vi "CRYAPI FRAME.vi"(4 "tFrame_In":T2, 6 "tSpliter":T3, 8 "tFrame":T2, 9 "sData":string, 10 "nData":i32, 11 "sAction":string) -> (0 "nData_Out":i32, 1 "sData_Out":string, 2 "tSpliter_Out":T3, 3 "tFrame_Out":T2)   [LabVIEW 2013]
uses:
  <vilib>/Utility/miscctls.llb/LVRectTypeDef.ctl
  CRYMain Sub Window Global.vi
  CRYProject/CRYProject Editor Global.vi
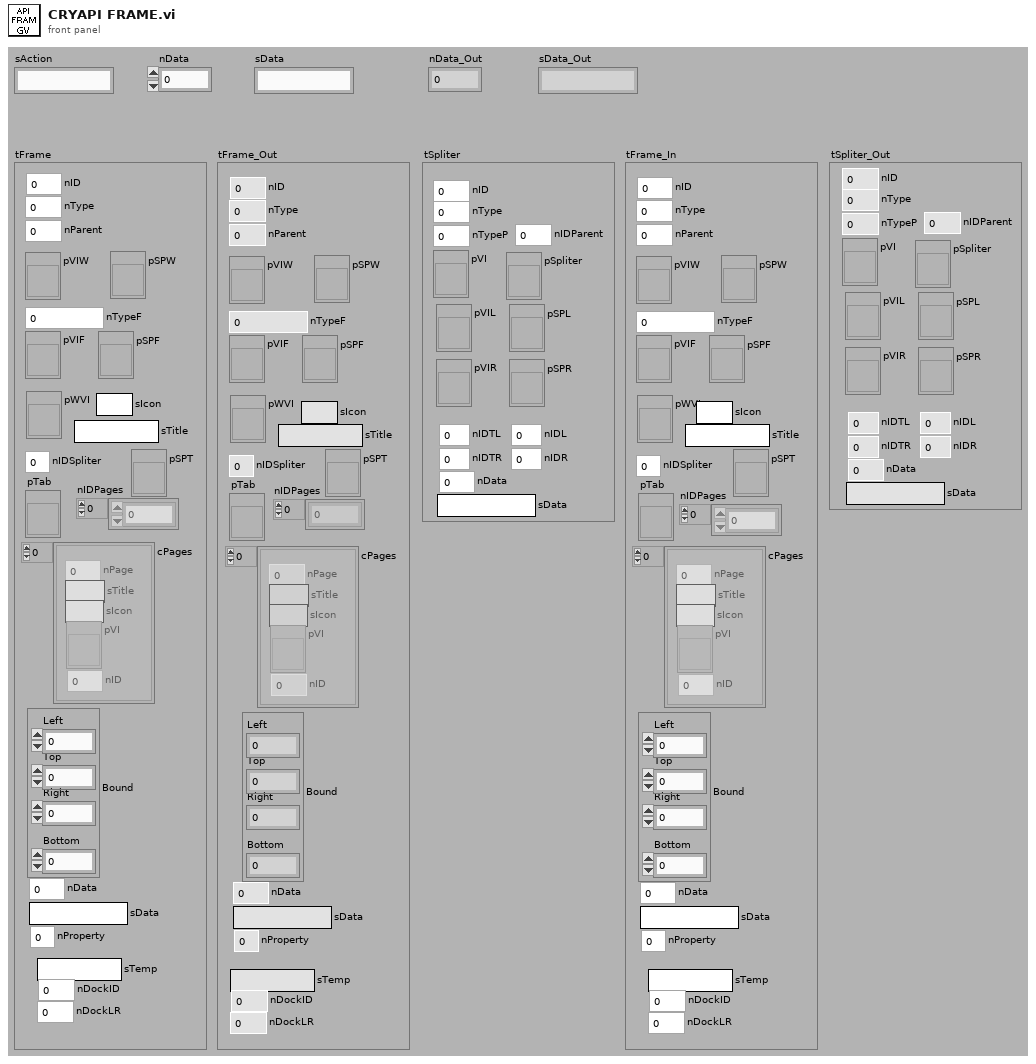
[diagram p1: front panel]
types:
  T1 = typedef "LVRectTypeDef.ctl" = cluster{"Left":i16, "Top":i16, "Right":i16, "Bottom":i16}
  T2 = cluster{"nType":i32, "nParent":i32, "pVIW":refnum<vi>, "pSPW":refnum<vi>, "nTypeF":i32, "pVIF":refnum<vi>, "pSPF":refnum<vi>, "nIDSpliter":i32, "nProperty":i32, "Bound":T1, "nID":i32, "nData":i32, "sData":string, "pWVI":refnum<vi>, "sTitle":string, "cPages":cluster{"nPage":i32, "sTitle":string, "sIcon":string, "pVI":refnum<vi>, "nID":i32}[], "pTab":refnum<vi>, "nIDPages":i32[], "pSPT":refnum<vi>, "sTemp":string, "nDockID":i32, "nDockLR":i32, "sIcon":string}
  T3 = cluster{"nType":i32, "nTypeP":i32, "pVI":refnum<vi>, "pSpliter":refnum<vi>, "pSPL":refnum<vi>, "pVIL":refnum<vi>, "pSPR":refnum<vi>, "pVIR":refnum<vi>, "nIDTL":i32, "nIDL":i32, "nIDTR":i32, "nIDR":i32, "nID":i32, "nIDParent":i32, "nData":i32, "sData":string}
  T4 = cluster{"nPage":i32, "sTitle":string, "sIcon":string, "pVI":refnum<vi>, "nID":i32}[]
  T5 = cluster{"nID":i32, "sTiltle":string, "pVI":refnum<vi>, "pSP":refnum<vi>, "pTab":refnum<vi>, "pSPT":refnum<vi>, "nWinType":i32, "sIcon":string}
  T6 = cluster{"nID":i32[], "Frame":cluster{"nType":i32, "nParent":i32, "pVIW":refnum<vi>, "pSPW":refnum<vi>, "nTypeF":i32, "pVIF":refnum<vi>, "pSPF":refnum<vi>, "nIDSpliter":i32, "nProperty":i32, "Bound":T1, "nID":i32, "nData":i32, "sData":string, "pWVI":refnum<vi>, "sTitle":string, "cPages":cluster{"nPage":i32, "sTitle":string, "sIcon":string, "pVI":refnum<vi>, "nID":i32}[], "pTab":refnum<vi>, "nIDPages":i32[], "pSPT":refnum<vi>, "sTemp":string, "nDockID":i32, "nDockLR":i32, "sIcon":string}[]}
  T7 = cluster{"nType":i32, "nParent":i32, "pVIW":refnum<vi>, "pSPW":refnum<vi>, "nTypeF":i32, "pVIF":refnum<vi>, "pSPF":refnum<vi>, "nIDSpliter":i32, "nProperty":i32, "Bound":T1, "nID":i32, "nData":i32, "sData":string, "pWVI":refnum<vi>, "sTitle":string, "cPages":cluster{"nPage":i32, "sTitle":string, "sIcon":string, "pVI":refnum<vi>, "nID":i32}[], "pTab":refnum<vi>, "nIDPages":i32[], "pSPT":refnum<vi>, "sTemp":string, "nDockID":i32, "nDockLR":i32, "sIcon":string}[]
  T8 = typedef "CRYTS.ctl" = cluster{"No.TS":u16, "TS File Path":path, "TS Name":string, "EditStepName":string, "Steps":T9[], "New State":bool, "Change State":bool, "Flattened CurveLib Data":string, "Document Data":string, "EditStepNo":u16, "Operator Start File":string, "Sequence Type":string, "Sequence Language":string}
  T9 = typedef "CRYStep.ctl" = cluster{"No.VI":i32, "Category":string, "StepName":string, "Seq setup flattened":string, "Comment":string, "Steps config.":bool[], "Jump config":i32[], "Start":dbl, "Increment":dbl, "Name":string, "Unit":string, "Y data":u16, "Y prefix":string, "Y dB ref":dbl, "Y unit":string, "Repeat State Array":cluster{"Start":dbl, "Increment":dbl, "Count":i32, "Num":i32}[]}
  T10 = typedef "LVPointTypeDef.ctl" = cluster{"Horizontal":i16, "Vertical":i16}
  T11 = typedef "LVBoundsTypeDef.ctl" = cluster{"Width":u32, "Height":u32}
  T12 = cluster{"nPage":i32, "sTitle":string, "sIcon":string, "pVI":refnum<vi>, "nID":i32}
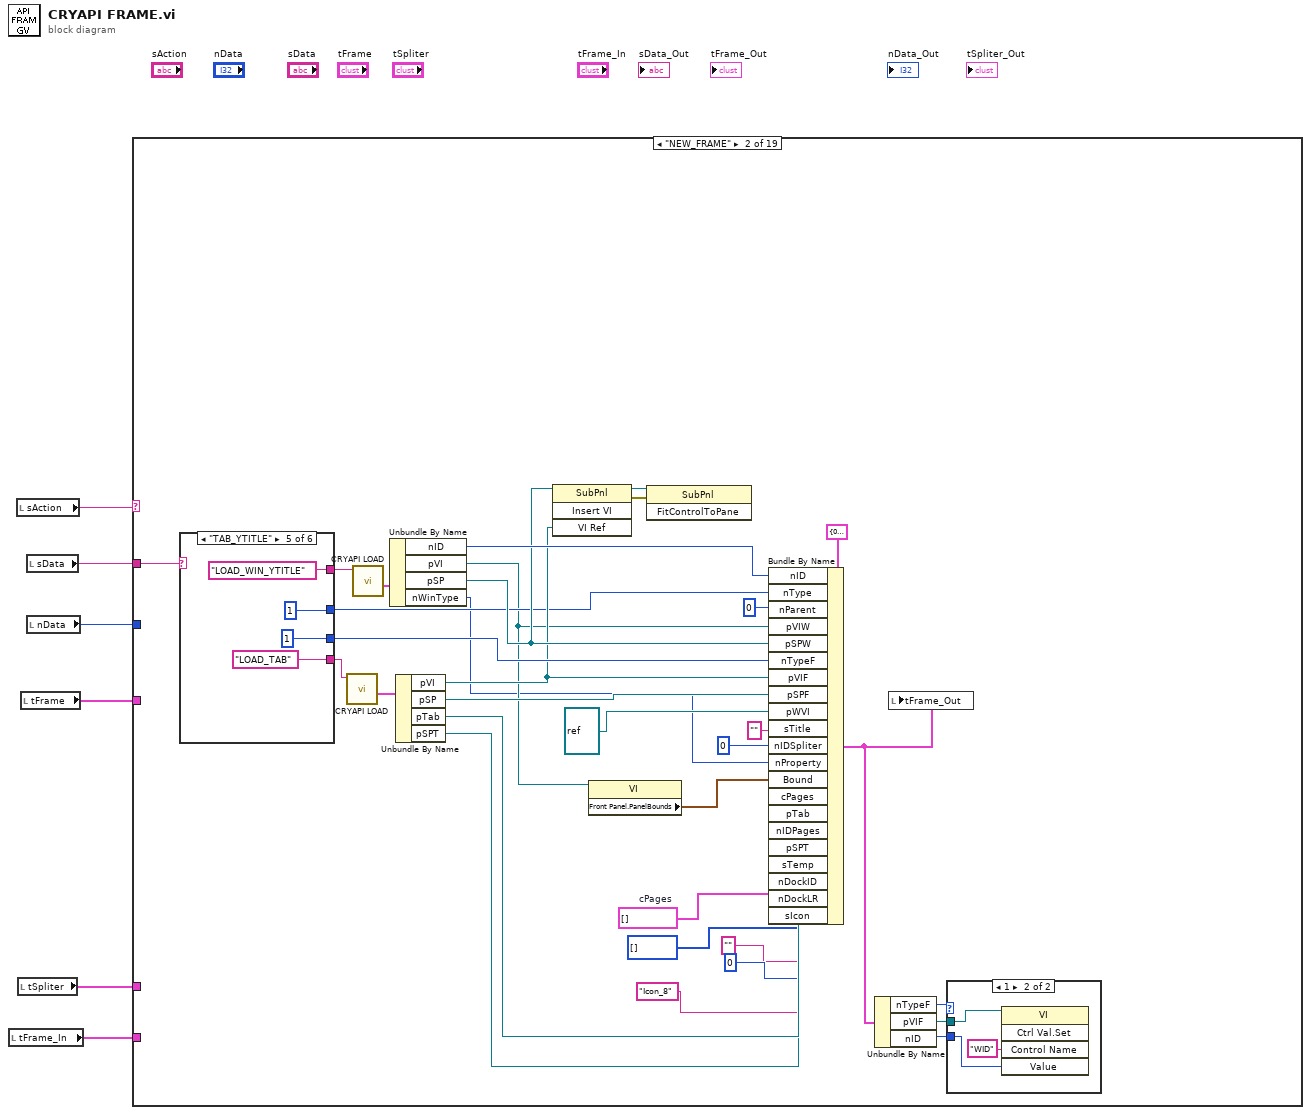
[diagram p0: block diagram]
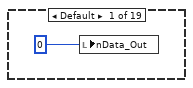
[diagram p2: hidden frame]
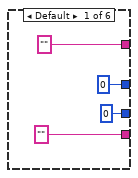
[diagram p4: hidden frame]
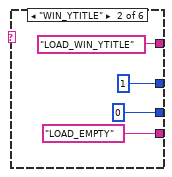
[diagram p5: hidden frame]
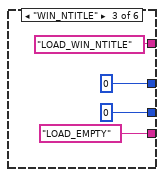
[diagram p6: hidden frame]
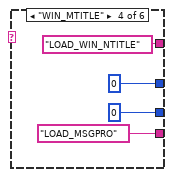
[diagram p7: hidden frame]
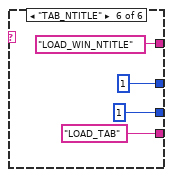
[diagram p8: hidden frame]
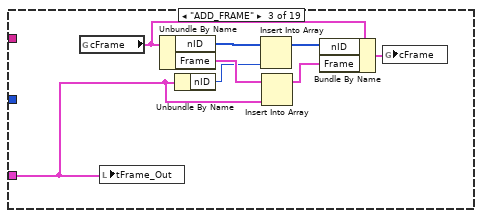
[diagram p9: hidden frame]
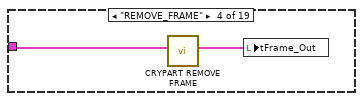
[diagram p10: hidden frame]
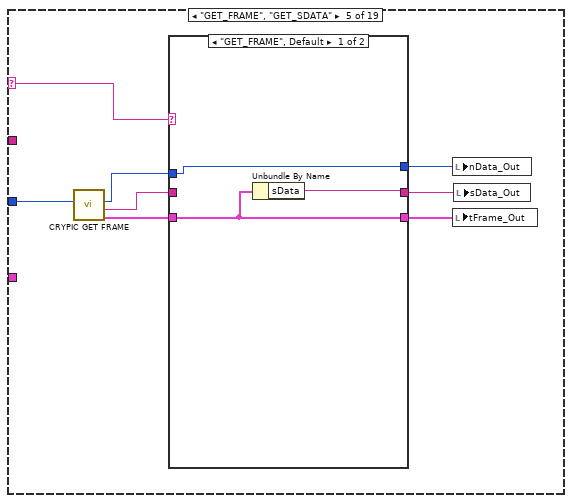
[diagram p11: hidden frame]
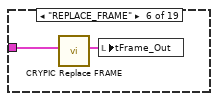
[diagram p13: hidden frame]
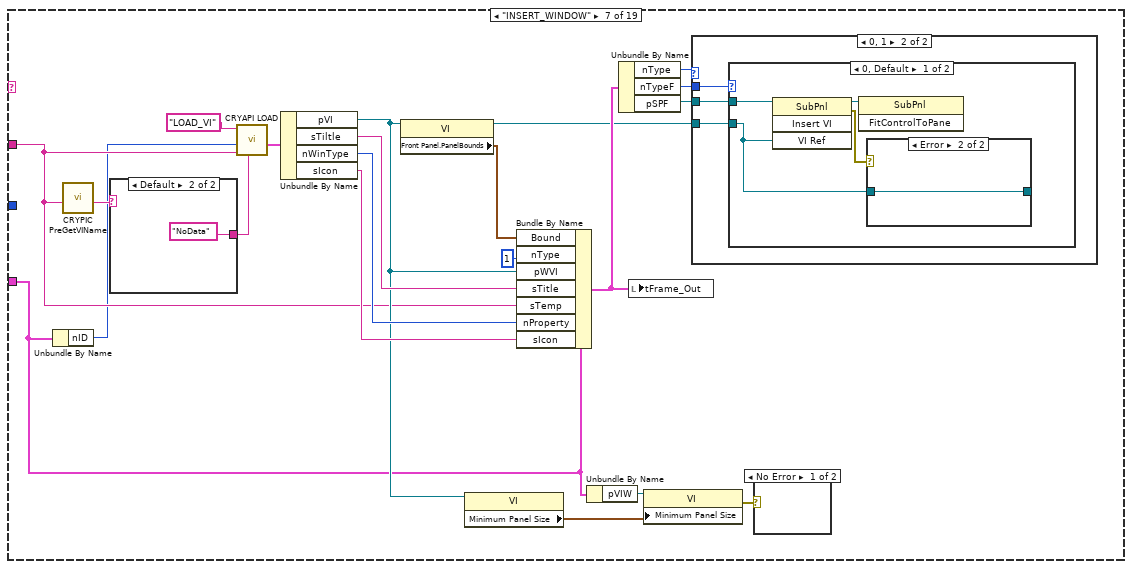
[diagram p14: hidden frame]
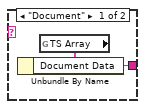
[diagram p16: hidden frame]
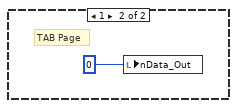
[diagram p19: hidden frame]
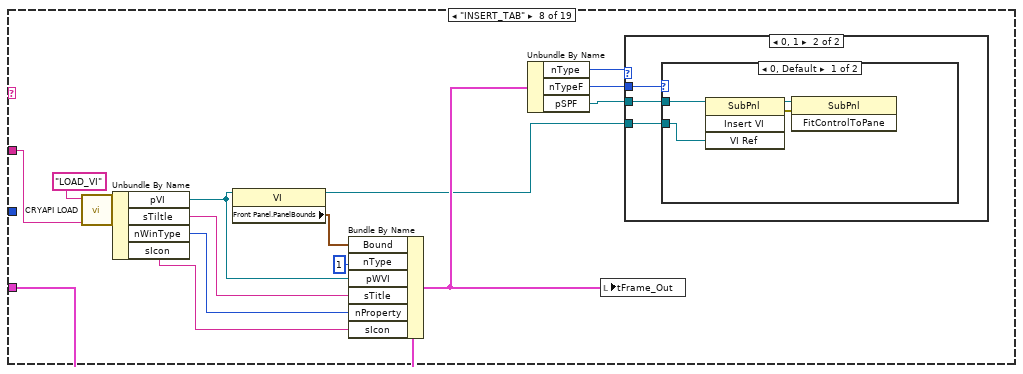
[diagram p20: hidden frame]
diagram:
  n1 = local read "tFrame_In"() -> (w1:T2)
  n2 = local read "sAction"() -> (w6:string)
  n3 = local read "tSpliter"() -> (w2:T3)
  n4 = local read "tFrame"() -> (w3:T2)
  n5 = local read "sData"() -> (w4:string)
  n6 = local read "nData"() -> (w5:i32)
  n7 = case shown="\"NEW_FRAME\"" w6 {
    selector: w6 -> [_ _ _ _ w80 _ _ _ _ w174 _ _ _ w378 w451 _ w569 _ _]
    tunnel: w5 -> [_ _ _ _ w84 _ _ _ _ _ _ _ _ _ _ w534 w568 _ _]
    tunnel: w4 -> [_ w19 _ _ _ _ w95 w139 _ _ _ _ _ _ _ _ w574 _ _]
    tunnel: w3 -> [_ _ w67 w76 _ w91 w94 w127 w163 w175 w300 w320 w348 w377 w452 w526 _ w628 w641]
    tunnel: w2 -> [_ _ _ _ _ _ _ _ w157 _ _ w319 w344 _ _ _ _ _ _]
    tunnel: w1 -> [_ _ _ _ _ _ _ _ _ w168 w302 _ _ _ _ _ _ _ _]
    frame Default {
      n8 = local write "nData_Out"(0 ("nData_Out")) -> ()
    }
    frame "NEW_FRAME" {
      w13 = 0 ("nIDChain")
      w26 = T4 []  # cPages
      n9 = case shown="\"TAB_YTITLE\"" w19 {
        tunnel: ["" ("sAction") "LOAD_WIN_YTITLE" ("sAction") "LOAD_WIN_NTITLE" ("sAction") "LOAD_WIN_NTITLE" ("sAction") "LOAD_WIN_YTITLE" ("sAction") "LOAD_WIN_NTITLE" ("sAction")] -> w12
        tunnel: ["" ("sAction") "LOAD_EMPTY" ("sAction") "LOAD_EMPTY" ("sAction") "LOAD_MSGPRO" ("sAction") "LOAD_TAB" ("sAction") "LOAD_TAB" ("sAction")] -> w18
        tunnel: [0 ("nTypeF") 0 ("nTypeF") 0 ("nTypeF") 0 ("nTypeF") 1 ("nTypeF") 1 ("nTypeF")] -> w34
        tunnel: [0 ("nTypeF") 1 ("nTypeF") 0 ("nTypeF") 0 ("nTypeF") 1 ("nTypeF") 1 ("nTypeF")] -> w29
        frame Default {
        }
        frame "WIN_YTITLE" {
        }
        frame "WIN_NTITLE" {
        }
        frame "WIN_MTITLE" {
        }
        frame "TAB_YTITLE" {
        }
        frame "TAB_NTITLE" {
        }
      }
      n10 = call "CRYAPI LOAD.vi"("sAction"=w18) -> ("tWindow_Out"=w17:T5)  [unwired: 5 in, 5 out]
      n11 = call "CRYAPI LOAD.vi"("sAction"=w12) -> ("tWindow_Out"=w37:T5)  [unwired: 5 in, 5 out]
      n12 = Unbundle By Name(w37) -> ("nID"=w36:i32, "pVI"=w15:refnum<vi>, "pSP"=w33:refnum<vi>, "nWinType"=w11:i32)
      n13 = Unbundle By Name(w17) -> ("pVI"=w32:refnum<vi>, "pSP"=w35:refnum<vi>, "pTab"=w25:refnum<vi>, "pSPT"=w16:refnum<vi>)
      n14 = invoke class="SubPnl" method="Insert VI"(reference=w33, "VI Ref"=w32) -> (reference out=w31:refnum<vi>, error out=w30:errorcluster)  [unwired: 2 in, 2 out]
      n15 = property class="VI"(reference=w15) -> ("Front Panel.PanelBounds"=w14:T1)  [unwired: 1 in, 2 out]
      n16 = invoke class="SubPnl" method="FitControlToPane"(reference=w31, error in=w30) -> ()  [unwired: 1 in, 3 out]
      n17 = Bundle By Name(cluster=T2 {"nType"=0, "nParent"=0, "pVIW"=refnum, "pSPW"=refnum, "nTypeF"=0, "pVIF"=refnum, "pSPF"=refnum, "nIDSpliter"=0, "nProperty"=0, "Bound"={"Left"=100, "Top"=100, "Right"=200, "Bottom"=200}, "nID"=0, "nData"=0, "sData"="", "pWVI"=refnum, "sTitle"="", "cPages"=[], "pTab"=refnum, "nIDPages"=[], "pSPT"=refnum, "sTemp"="", "nDockID"=0, "nDockLR"=0, "sIcon"=""} ("tFrame_Out"), "nID"=w36, "nType"=w29, "nParent"=0, "pVIW"=w15, "pSPW"=w33, "nTypeF"=w34, "pVIF"=w32, "pSPF"=w35, "pWVI"=refnum<vi> refnum, "sTitle"="", "nIDSpliter"=0 ("nIDChain"), "nProperty"=w11, "Bound"=w14, "cPages"=w26, "pTab"=w25, "nIDPages"=i32[] [], "pSPT"=w16, "sTemp"="", "nDockID"=w13, "nDockLR"=w13, "sIcon"="Icon_8") -> (w24:T2)
      n18 = Unbundle By Name(w24) -> ("nTypeF"=w23:i32, "pVIF"=w22:refnum<vi>, "nID"=w21:i32)
      n19 = local write "tFrame_Out"(w24) -> ()
      n20 = case shown="1" w23 {
        tunnel: w22 -> [_ w42]
        tunnel: w21 -> [_ w40]
        frame Default {
        }
        frame 1 {
          n21 = invoke class="VI" method="Ctrl Val.Set"(reference=w42, "Control Name"="WID", "Value"=w40) -> ()  [unwired: 2 in, 5 out]
        }
      }
    }
    frame "ADD_FRAME" {
      n22 = global read "CRYMain Sub Window Global.vi" "cFrame"() -> (w71:T6)
      n23 = local write "tFrame_Out"(w67) -> ()
      n24 = Unbundle By Name(w71) -> ("nID"=w74:i32[], "Frame"=w73:T7)
      n25 = Unbundle By Name(w67) -> ("nID"=w72:i32)
      n26 = Insert Into Array(array=w74, new element=w72) -> (w70:i32[])  [unwired: 1 in]
      n27 = Insert Into Array(array=w73, new element=w67) -> (w69:T7)  [unwired: 1 in]
      n28 = Bundle By Name(cluster=w71, "nID"=w70, "Frame"=w69) -> (w68:T6)
      n29 = global write "CRYMain Sub Window Global.vi" "cFrame"(w68) -> ()
    }
    frame "REMOVE_FRAME" {
      n30 = call "CRYPART REMOVE FRAME.vi"("tFrame"=w76) -> ("tFrame_Out"=w75:T2)  [unwired: 10 in]
      n31 = local write "tFrame_Out"(w75) -> ()
    }
    frame "GET_FRAME", "GET_SDATA" {
      n32 = call "CRYPIC GET FRAME.vi"("nID"=w84) -> ("tFrame_Out"=w81:T2, "sData_Out"=w82:string, "nID_Out"=w83:i32)  [unwired: 8 in]
      n33 = case shown="\"GET_FRAME\", Default" w80 {
        tunnel: w83 -> [w87 w90]
        tunnel: w82 -> [_ w88]
        tunnel: w81 -> [w86 w89]
        tunnel: [w87 w90] -> w79
        tunnel: [w85 w88] -> w78
        tunnel: [w86 w89] -> w77
        frame "GET_FRAME", Default {
          n34 = Unbundle By Name(w86) -> ("sData"=w85:string)
        }
        frame "GET_SDATA" {
        }
      }
      n35 = local write "nData_Out"(w79) -> ()
      n36 = local write "tFrame_Out"(w77) -> ()
      n37 = local write "sData_Out"(w78) -> ()
    }
    frame "REPLACE_FRAME" {
      n38 = call "CRYPIC Replace FRAME.vi"("tFrame"=w91) -> ("tFrame_Out"=w92:T2)  [unwired: 10 in]
      n39 = local write "tFrame_Out"(w92) -> ()
    }
    frame "INSERT_WINDOW" {
      n40 = Unbundle By Name(w94) -> ("nID"=w93:i32)
      n41 = call "CRYPIC PreGetVIName.vi"("sVIName"=w95) -> ("sVIName_Out"=w96:string)  [unwired: 9 in, 1 out]
      n42 = case shown="Default" w96 {
        tunnel: [w114 "NoData" ("sOption")] -> w101
        frame "Document" {
          n43 = global read "CRYProject Editor Global.vi" "TS Array"() -> (w115:T8)
          n44 = Unbundle By Name(w115) -> ("Document Data"=w114:string)
        }
        frame Default {
        }
      }
      n45 = call "CRYAPI LOAD.vi"("sOption"=w101, "sData"=w95, "nData"=w93, "sAction"="LOAD_VI") -> ("tWindow_Out"=w103:T5)  [unwired: 2 in, 5 out]
      n46 = Unbundle By Name(w103) -> ("pVI"=w98:refnum<vi>, "sTiltle"=w106:string, "nWinType"=w105:i32, "sIcon"=w104:string)
      n47 = property class="VI"(reference=w98) -> (reference out=w109:refnum<vi>, "Front Panel.PanelBounds"=w112:T1)  [unwired: 1 in, 1 out]
      n48 = property class="VI"(reference=w98) -> ("Minimum Panel Size"=w99:T10)  [unwired: 1 in, 2 out]
      n49 = Bundle By Name(cluster=w94, "Bound"=w112, "nType"=1, "pWVI"=w98, "sTitle"=w106, "sTemp"=w95, "nProperty"=w105, "sIcon"=w104) -> (w111:T2)
      n50 = Unbundle By Name(w94) -> ("pVIW"=w100:refnum<vi>)
      n51 = Unbundle By Name(w111) -> ("nType"=w110:i32, "nTypeF"=w108:i32, "pSPF"=w107:refnum<vi>)
      n52 = local write "tFrame_Out"(w111) -> ()
      n53 = property class="VI"(reference=w100, "Minimum Panel Size"=w99) -> (error out=w97:errorcluster)  [unwired: 1 in, 1 out]
      n54 = case shown="0, 1" w110 {
        tunnel: w109 -> [_ w117]
        tunnel: w108 -> [_ w119]
        tunnel: w107 -> [_ w118]
        frame Default {
        }
        frame 0, 1 {
          n55 = case shown="0, Default" w119 {
            tunnel: w118 -> [w122 _]
            tunnel: w117 -> [w120 _]
            frame 0, Default {
              n56 = invoke class="SubPnl" method="Insert VI"(reference=w122, "VI Ref"=w120) -> (reference out=w123:refnum<vi>, error out=w121:errorcluster)  [unwired: 2 in, 2 out]
              n57 = invoke class="SubPnl" method="FitControlToPane"(reference=w123) -> ()  [unwired: 2 in, 3 out]
              n58 = case shown="Error" w121 {
                tunnel: [w124 w125] -> _
                tunnel: w120 -> [w124 w125]
                frame No Error {
                }
                frame Error {
                }
              }
            }
            frame 1 {
              # "TAB Page"
              n59 = local write "nData_Out"(0 ("nData_Out")) -> ()
            }
          }
        }
      }
      n60 = case shown="No Error" w97 {
        frame No Error {
        }
        frame Error {
        }
      }
    }
    frame "INSERT_TAB" {
      n61 = call "CRYAPI LOAD.vi"("sData"=w139, "sAction"="LOAD_VI") -> ("tWindow_Out"=w140:T5)  [unwired: 4 in, 5 out]
      n62 = Unbundle By Name(w140) -> ("pVI"=w132:refnum<vi>, "sTiltle"=w131:string, "nWinType"=w130:i32, "sIcon"=w129:string)
      n63 = property class="VI"(reference=w132) -> (reference out=w128:refnum<vi>, "Front Panel.PanelBounds"=w137:T1)  [unwired: 1 in, 1 out]
      n64 = Bundle By Name(cluster=w127, "Bound"=w137, "nType"=1, "pWVI"=w132, "sTitle"=w131, "nProperty"=w130, "sIcon"=w129) -> (w136:T2)
      n65 = Unbundle By Name(w136) -> ("nType"=w135:i32, "nTypeF"=w134:i32, "pSPF"=w133:refnum<vi>)
      n66 = local write "tFrame_Out"(w136) -> ()
      n67 = case shown="0, 1" w135 {
        tunnel: w128 -> [_ w142]
        tunnel: w134 -> [_ w144]
        tunnel: w133 -> [_ w143]
        frame Default {
        }
        frame 0, 1 {
          n68 = case shown="0, Default" w144 {
            tunnel: w143 -> [w146 _]
            tunnel: w142 -> [w145 _]
            frame 0, Default {
              n69 = invoke class="SubPnl" method="Insert VI"(reference=w146, "VI Ref"=w145) -> (reference out=w148:refnum<vi>, error out=w147:errorcluster)  [unwired: 2 in, 2 out]
              n70 = invoke class="SubPnl" method="FitControlToPane"(reference=w148, error in=w147) -> ()  [unwired: 1 in, 3 out]
            }
            frame 1 {
              # "TAB Page"
              n71 = local write "nData_Out"(0 ("nData_Out")) -> ()
            }
          }
        }
      }
    }
    frame "INSERT_SPLITER" {
      n72 = Unbundle By Name(w163) -> ("pSPF"=w151:refnum<vi>, "nType"=w150:i32, "nID"=w156:i32)
      n73 = case shown="0" w150 {
        tunnel: [0 ("nParent") 2 ("nType")] -> w152
        frame 0 {
        }
        frame Default {
        }
      }
      n74 = Bundle By Name(cluster=w157, "nIDParent"=w156, "nTypeP"=0 ("nParent")) -> (w154:T3)
      n75 = Unbundle By Name(w157) -> ("pVI"=w162:refnum<vi>, "nID"=w161:i32)
      n76 = Bundle By Name(cluster=w163, "nIDSpliter"=w161, "nType"=w152) -> (w158:T2)
      n77 = invoke class="SubPnl" method="Insert VI"(reference=w151, "VI Ref"=w162) -> (reference out=w160:refnum<vi>, error out=w159:errorcluster)  [unwired: 2 in, 2 out]
      n78 = call "CRYAPI SPLITE.vi"("tSpliter"=w154, "sAction"="REPLACE_SPLITER") -> ()  [unwired: 4 in, 6 out]
      n79 = local write "tFrame_Out"(w158) -> ()
      n80 = invoke class="SubPnl" method="FitControlToPane"(reference=w160, error in=w159) -> ()  [unwired: 1 in, 3 out]
    }
    frame "SET_DOCK", "SET_FRAME", "SET_FRAME_CLONE" {
      n81 = Unbundle By Name(w175) -> ("nType"=w177:i32, "pVIW"=w176:refnum<vi>, "nID"=w178:i32, "nParent"=w173:i32, "sTitle"=w172:string, "nTypeF"=w171:i32, "Bound"=w170:T1, "pVIW"=w169:refnum<vi>, "nProperty"=w167:i32, "sIcon"=w166:string)
      n82 = case shown="\"SET_FRAME\"" w174 {
        tunnel: w177 -> [_ w185 w202 _]
        tunnel: w176 -> [_ w184 w204 w269]
        tunnel: w175 -> [_ w180 w195 w289]
        tunnel: w178 -> [_ _ w208 w296]
        tunnel: w173 -> [_ w181 w201 w293]
        tunnel: w172 -> [_ _ w207 _]
        tunnel: w171 -> [_ _ w206 w273]
        tunnel: w170 -> [_ _ _ _]
        tunnel: w169 -> [_ _ _ w285]
        tunnel: w168 -> [_ _ _ w287]
        tunnel: w167 -> [_ _ w203 _]
        tunnel: w166 -> [_ _ w200 _]
        frame Default {
          n83 = local write "nData_Out"(0 ("nData_Out")) -> ()
        }
        frame "SET_DOCK" {
          n84 = local write "tFrame_Out"(w180) -> ()
          n85 = Not Equal?(x=w181, y=0) -> (x != y?=w182:bool)
          n86 = case shown="Default" w185 {
            tunnel: w184 -> [_ w188]
            tunnel: w182 -> [_ w187]
            tunnel: w180 -> [_ w186]
            frame 0 {
            }
            frame Default {
              n87 = case shown="False" w187 {
                tunnel: w188 -> [w190 w193]
                tunnel: w186 -> [_ _]
                frame True {
                  n88 = invoke class="VI" method="Ctrl Val.Set"(reference=w190, "Control Name"="DockState", "Value"=TRUE ("bResult")) -> ()  [unwired: 2 in, 5 out]
                }
                frame False {
                  n89 = invoke class="VI" method="Ctrl Val.Set"(reference=w193, "Control Name"="DockState", "Value"=FALSE ("bResult")) -> ()  [unwired: 2 in, 5 out]
                }
              }
            }
          }
        }
        frame "SET_FRAME" {
          n90 = case shown="1" w202 {
            selector: w202 -> [_ w247 w259]
            tunnel: w204 -> [_ w245 w256]
            tunnel: w207 -> [_ _ w257]
            tunnel: w206 -> [_ _ w263]
            tunnel: ["NO TITLE" ("Control Name") w248 w250] -> w196
            tunnel: w200 -> [_ w244 w258]
            tunnel: [_ w247 w259] -> w199
            tunnel: [_ w246 w255] -> w198
            tunnel: [_ w244 w258] -> w197
            frame Default {
            }
            frame 2 {
              w248 = "" ("Control Name")
              # "FRAME"
              n91 = invoke class="VI" method="Ctrl Val.Set"(reference=w245, "Control Name"="TitleName", "Value"=w248) -> (reference out=w246:refnum<vi>)  [unwired: 2 in, 4 out]
            }
            frame 1 {
              # "TAB"
              n92 = Equal?(x=w263, y=0) -> (x = y?=w261:bool)
              n93 = Select(t=w257, s=w261, f="" ("Control Name")) -> (s? t:f=w250:string)
              n94 = call "CRYGet Boolean Reference.vi"("Label Name"="bTitleChange" ("Control Name"), "VI Refnum"=w256) -> ("Boolean Ref"=w251:refnum<vi>, "VI Refnum Out"=w255:refnum<vi>)  [unwired: 7 in, 1 out]
              n95 = Build Array(w250) -> (w253:string[])
              n96 = call "CRYDisplay Unicode Boolean Text.vi"("Interpret as Unicode (T)"=TRUE, "Boolean Texts [4]"=w253, "Boolean Reference"=w251) -> ()  [unwired: 5 in, 2 out]
            }
          }
          n97 = case shown="1, 2" w202 {
            tunnel: w208 -> [_ w242]
            tunnel: w201 -> [_ w235]
            tunnel: w204 -> [_ w237]
            tunnel: w203 -> [_ w236]
            frame 0, Default {
            }
            frame 1, 2 {
              n98 = Not Equal To 0?(x=w235) -> (x != 0?=w239:bool)
              n99 = invoke class="VI" method="Ctrl Val.Set"(reference=w237, "Control Name"="WindowNumber", "Value"=w242) -> ()  [unwired: 2 in, 5 out]
              n100 = invoke class="VI" method="Ctrl Val.Set"(reference=w237, "Control Name"="nWinType", "Value"=w236) -> ()  [unwired: 2 in, 5 out]
              n101 = invoke class="VI" method="Ctrl Val.Set"(reference=w237, "Control Name"="DockState", "Value"=w239) -> ()  [unwired: 2 in, 5 out]
            }
          }
          n102 = Bundle By Name(cluster=w195, "sTitle"=w196) -> (w205:T2)
          n103 = case shown="1, 2" w199 {
            tunnel: w198 -> [_ w231]
            tunnel: w197 -> [_ w233]
            tunnel: w196 -> [_ w225]
            frame 0, Default {
            }
            frame 1, 2 {
              n104 = Search/Split String(string=w233, search string/char (-)="_" ("search string")) -> (match + rest of string=w230:string)  [unwired: 3 out]
              n105 = String Subset(string=w230, offset (0)=1) -> (substring=w228:string)  [unwired: 1 out]
              n106 = Empty String/Path?(string/path=w225) -> (empty?=w224:bool)
              n107 = Decimal String To Number(string=w228) -> (number=w227:i32)  [unwired: 3 out]
              n108 = Not(x=w224) -> (.not. x?=w223:bool)
              n109 = Decrement(x=w227) -> (x-1=w226:i32)
              n110 = Select(t=w226, s=w223, f=7) -> (s? t:f=w221:i32)
              n111 = invoke class="VI" method="Ctrl Val.Set"(reference=w231, "Control Name"="IconRing", "Value"=w221) -> ()  [unwired: 2 in, 5 out]
            }
          }
          n112 = flat-sequence {
            tunnel: w195 -> [w210]
            frame #0 {
              n113 = Unbundle By Name(w210) -> ("pVIW"=w212:refnum<vi>, "pWVI"=w218:refnum<vi>, "nID"=w211:i32)
              n114 = property class="VI"(reference=w218) -> (error out=w209:errorcluster, "Minimum Panel Size"=w213:T10)  [unwired: 1 in, 1 out]
              n115 = call "CRYGet Numeric Reference.vi"("Label Name"="nIDFParent", "VI Refnum"=w218) -> ("Boolean"=w216:bool, "Numeric Ref Out"=w217:refnum<vi>)  [unwired: 7 in, 1 out]
              n116 = case shown="True" w216 {
                tunnel: w217 -> [_ w220]
                tunnel: w211 -> [_ w219]
                frame False {
                }
                frame True {
                  n117 = property class="DigNum"(reference=w220, "Value"=w219) -> ()  [unwired: 1 in, 2 out]
                }
              }
              n118 = property class="VI"(reference=w212, error in=w209, "Minimum Panel Size"=w213) -> (error out=w214:errorcluster)  [unwired: 1 out]
              n119 = case shown="No Error" w214 {
                frame No Error {
                }
                frame Error {
                }
              }
            }
          }
          n120 = local write "tFrame_Out"(w205) -> ()
        }
        frame "SET_FRAME_CLONE" {
          # "TAB"
          # "FRAME"
          n121 = Equal?(x=w273, y=0) -> (x = y?=w282:bool)
          n122 = Select(t=2 ("y"), s=w282, f=1 ("y")) -> (s? t:f=w278:i32)
          n123 = Unbundle By Name(w287) -> ("pVIW"=w286:refnum<vi>, "nParent"=w283:i32)
          n124 = Not Equal?(x=w293, y=0) -> (x != y?=w291:bool)
          n125 = local write "nData_Out"(w283) -> ()
          n126 = property class="VI"(reference=w286) -> ("Front Panel.PanelBounds"=w284:T1)  [unwired: 1 in, 2 out]
          n127 = invoke class="VI" method="Ctrl Val.Set"(reference=w269, "Control Name"="WindowNumber", "Value"=w296) -> ()  [unwired: 2 in, 5 out]
          n128 = invoke class="VI" method="Ctrl Val.Set"(reference=w269, "Control Name"="DockState", "Value"=w291) -> ()  [unwired: 2 in, 5 out]
          n129 = invoke class="VI" method="Ctrl Val.Set"(reference=w269, "Control Name"="nWinType", "Value"=0 ("y")) -> ()  [unwired: 2 in, 5 out]
          n130 = Equal?(x=w273, y=0) -> (x = y?=w276:bool)
          n131 = Select(t="" ("Control Name"), s=w276, f="" ("Control Name")) -> (s? t:f=w272:string)
          n132 = property class="VI"(reference=w285, "Front Panel.PanelBounds"=w284) -> (error out=w264:errorcluster)  [unwired: 1 in, 1 out]
          n133 = Bundle By Name(cluster=w289, "sTitle"=w272, "nType"=w278, "Bound"=w284, "nParent"=w283, "nProperty"=0) -> (w288:T2)
          n134 = invoke class="VI" method="Ctrl Val.Set"(reference=w269, "Control Name"="TitleName", "Value"=w272) -> (reference out=w267:refnum<vi>)  [unwired: 2 in, 4 out]
          n135 = local write "tFrame_Out"(w288) -> ()
          n136 = case shown="No Error" w264 {
            frame No Error {
            }
            frame Error {
            }
          }
          n137 = invoke class="VI" method="Ctrl Val.Set"(reference=w267, "Control Name"="IconRing", "Value"=7) -> ()  [unwired: 2 in, 5 out]
        }
      }
    }
    frame "CLONE_FRAME" {
      n138 = Unbundle By Name(w302) -> ("pVIW"=w301:refnum<vi>)
      n139 = property class="VI"(reference=w301) -> ("Front Panel.PanelBounds"=w297:T1)  [unwired: 1 in, 2 out]
      n140 = Bundle By Name(cluster=w300, "nType"=2, "Bound"=w297) -> (w298:T2)
      n141 = local write "tFrame_Out"(w298) -> ()
    }
    frame "INSERT_COMPLETE" {
      w305 = "ActiveNumber" ("Control Name")
      n142 = Unbundle By Name(w320) -> ("pSPF"=w310:refnum<vi>, "nType"=w330:i32, "nID"=w325:i32, "pVIW"=w308:refnum<vi>)
      n143 = case shown="Default" w330 {
        tunnel: [0 ("nParent") 2 ("nType")] -> w329
        frame 0 {
        }
        frame Default {
        }
      }
      n144 = Bundle By Name(cluster=w319, "nIDParent"=w325, "nTypeP"=0 ("nParent")) -> (w327:T3)
      n145 = Unbundle By Name(w319) -> ("nID"=w321:i32)
      n146 = Bundle By Name(cluster=w320, "nIDSpliter"=w321, "nType"=w329) -> (w324:T2)
      n147 = invoke class="VI" method="Ctrl Val.Get"(reference=w308, "Control Name"=w305) -> ("Get Control Value Variant"=w307:variant)  [unwired: 2 in, 3 out]
      n148 = call "CRYAPI SPLITE.vi"("tSpliter"=w327, "sAction"="REPLACE_SPLITER") -> ("tSpliter_Out"=w318:T3)  [unwired: 4 in, 5 out]
      n149 = local write "tFrame_Out"(w324) -> ()
      n150 = Unbundle By Name(w318) -> ("pVI"=w317:refnum<vi>, "pSPL"=w315:refnum<vi>, "pVIL"=w309:refnum<vi>, "pSPR"=w311:refnum<vi>, "pVIR"=w306:refnum<vi>, "nIDTL"=w304:i32, "nIDTR"=w303:i32)
      n151 = invoke class="SubPnl" method="Insert VI"(reference=w310, "VI Ref"=w317) -> (reference out=w322:refnum<vi>, error out=w323:errorcluster)  [unwired: 2 in, 2 out]
      n152 = invoke class="SubPnl" method="Insert VI"(reference=w315, "VI Ref"=w309) -> (reference out=w316:refnum<vi>, error out=w314:errorcluster)  [unwired: 2 in, 2 out]
      n153 = invoke class="SubPnl" method="Insert VI"(reference=w311, "VI Ref"=w306) -> (reference out=w312:refnum<vi>, error out=w313:errorcluster)  [unwired: 2 in, 2 out]
      n154 = case shown="0" w304 {
        tunnel: w309 -> [_ w336]
        tunnel: w307 -> [_ w335]
        tunnel: w305 -> [_ w334]
        frame Default {
        }
        frame 0 {
          n155 = invoke class="VI" method="Ctrl Val.Set"(reference=w336, "Control Name"=w334, "Value"=w335) -> ()  [unwired: 2 in, 5 out]
        }
      }
      n156 = case shown="0" w303 {
        tunnel: w307 -> [_ w333]
        tunnel: w306 -> [_ w332]
        tunnel: w305 -> [_ w331]
        frame Default {
        }
        frame 0 {
          n157 = invoke class="VI" method="Ctrl Val.Set"(reference=w332, "Control Name"=w331, "Value"=w333) -> ()  [unwired: 2 in, 5 out]
        }
      }
      n158 = invoke class="SubPnl" method="FitControlToPane"(reference=w322, error in=w323) -> ()  [unwired: 1 in, 3 out]
      n159 = invoke class="SubPnl" method="FitControlToPane"(reference=w316, error in=w314) -> ()  [unwired: 1 in, 3 out]
      n160 = invoke class="SubPnl" method="FitControlToPane"(reference=w312, error in=w313) -> ()  [unwired: 1 in, 3 out]
    }
    frame "EXCHANGE_PARENT" {
      n161 = Unbundle By Name(w348) -> ("nParent"=w354:i32)
      n162 = call "CRYAPI SPLITE.vi"("nData"=w354, "sAction"="GET_SPLITER") -> ("tSpliter_Out"=w349:T3)  [unwired: 4 in, 5 out]
      n163 = Bundle By Name(cluster=w344, "nIDParent"=w354, "nTypeP"=1) -> (w351:T3)
      n164 = Unbundle By Name(w344) -> ("pVI"=w343:refnum<vi>, "nID"=w342:i32)
      n165 = call "CRYAPI SPLITE.vi"("tFrame"=w348, "tSpliter"=w349, "sAction"="GET_FRAME_LR") -> ("nData_Out"=w346:i32, "tSpliter_Out"=w347:T3)  [unwired: 3 in, 4 out]
      n166 = case shown="0, 1, Default" w346 {
        selector: w346 -> [w357 w363]
        tunnel: w347 -> [w361 w368]
        tunnel: [w362 w369] -> w345
        tunnel: [w360 w367] -> w340
        tunnel: w343 -> [w359 w366]
        tunnel: w342 -> [w358 w365]
        frame 0, 1, Default {
          n167 = Unbundle By Name(w361) -> ("pSPL"=w362:refnum<vi>)
          n168 = Bundle By Name(cluster=w361, "pVIL"=w359, "nIDL"=w358, "nData"=w357, "nIDTL"=1) -> (w360:T3)
        }
        frame 2 {
          n169 = Unbundle By Name(w368) -> ("pSPR"=w369:refnum<vi>)
          n170 = Bundle By Name(cluster=w368, "pVIR"=w366, "nIDR"=w365, "nData"=w363, "nIDTR"=1) -> (w367:T3)
        }
      }
      n171 = call "CRYAPI SPLITE.vi"("tSpliter"=w351, "sAction"="REPLACE_SPLITER") -> ()  [unwired: 4 in, 6 out]
      n172 = invoke class="SubPnl" method="Remove VI"(reference=w345) -> ()  [unwired: 2 in, 3 out]
      n173 = call "CRYAPI SPLITE.vi"("tSpliter"=w340, "sAction"="REPLACE_SPLITER") -> ("tSpliter_Out"=w339:T3)  [unwired: 4 in, 5 out]
      n174 = local write "tSpliter_Out"(w339) -> ()
    }
    frame "FLOAT_FRAME", "FLOAT_FRAME_HIDE" {
      n175 = Unbundle By Name(w377) -> ("nParent"=w395:i32, "pVIW"=w388:refnum<vi>, "Bound"=w389:T1)
      n176 = Unbundle By Name(w389) -> ("Right"=w387:i16, "Left"=w386:i16, "Bottom"=w385:i16, "Top"=w384:i16)
      n177 = Subtract(x=w387, y=w386) -> (x-y=w383:i16)
      n178 = Subtract(x=w385, y=w384) -> (x-y=w382:i16)
      n179 = call "CRYAPI SPLITE.vi"("nData"=w395, "sAction"="GET_SPLITER") -> ("tSpliter_Out"=w381:T3)  [unwired: 4 in, 5 out]
      n180 = Unbundle By Name(w381) -> ("pVI"=w391:refnum<vi>)
      n181 = property class="VI"(reference=w391) -> ("Front Panel.PanelBounds"=w390:T1)  [unwired: 1 in, 2 out]
      n182 = call "CRYAPI SPLITE.vi"("tFrame"=w377, "tSpliter"=w381, "sAction"="GET_FRAME_LR") -> ("nData_Out"=w392:i32, "tSpliter_Out"=w397:T3)  [unwired: 3 in, 4 out]
      n183 = case shown="2" w392 {
        tunnel: w397 -> [w447 w449]
        tunnel: [w448 w450] -> w380
        frame 0, 1, Default {
          n184 = Unbundle By Name(w447) -> ("pSPL"=w448:refnum<vi>)
        }
        frame 2 {
          n185 = Unbundle By Name(w449) -> ("pSPR"=w450:refnum<vi>)
        }
      }
      n186 = Unbundle By Name(w377) -> ("sTemp"=w376:string, "pSPF"=w375:refnum<vi>)
      n187 = property class="SubPnl"(reference=w380) -> ("Bounds"=w379:T11)  [unwired: 1 in, 2 out]
      n188 = case shown="2" w392 {
        tunnel: w390 -> [w408 w426]
        tunnel: w388 -> [w407 w425]
        tunnel: [w407 w425] -> w370
        tunnel: [w406 w424] -> _
        tunnel: w383 -> [w405 w423]
        tunnel: w382 -> [w404 w422]
        tunnel: w379 -> [_ w421]
        frame 0, 1, Default {
          n189 = Unbundle By Name(w408) -> ("Left"=w412:i16, "Top"=w411:i16)
          n190 = Add(x=w412, y=w405) -> (x+y=w410:i16)
          n191 = Add(x=w411, y=w404) -> (x+y=w409:i16)
          n192 = Bundle By Name(cluster=w408, "Left"=w412, "Top"=w411, "Right"=w410, "Bottom"=w409) -> (w406:T1)
        }
        frame 2 {
          n193 = Unbundle By Name(w426) -> ("Right"=w418:i16, "Bottom"=w420:i16)
          n194 = Unbundle By Name(w421) -> ("Width"=w417:u32, "Height"=w419:u32)
          n195 = Subtract(x=w418, y=w417) -> (x-y=w416:u32)
          n196 = Subtract(x=w420, y=w419) -> (x-y=w415:u32)
          n197 = Add(x=w416, y=w423) -> (x+y=w413:u32)
          n198 = Add(x=w415, y=w422) -> (x+y=w414:u32)
          n199 = Bundle By Name(cluster=w426, "Left"=w416, "Top"=w415, "Right"=w413, "Bottom"=w414) -> (w424:T1)
        }
      }
      n200 = case shown="\"Document\"" w376 {
        tunnel: [w401 w403] -> w393
        tunnel: w380 -> [w400 w402]
        tunnel: w375 -> [w399 _]
        frame "Document" {
          n201 = invoke class="SubPnl" method="Remove VI"(reference=w399) -> (error out=w398:errorcluster)  [unwired: 2 in, 2 out]
          n202 = invoke class="SubPnl" method="Remove VI"(reference=w400, error in=w398) -> (error out=w401:errorcluster)  [unwired: 1 in, 2 out]
        }
        frame Default {
          n203 = invoke class="SubPnl" method="Remove VI"(reference=w402) -> (error out=w403:errorcluster)  [unwired: 2 in, 2 out]
        }
      }
      n204 = local read "tFrame"() -> (w374:T2)
      n205 = Unbundle By Name(w374) -> ("sTemp"=w373:string, "pSPF"=w372:refnum<vi>, "pWVI"=w371:refnum<vi>)
      n206 = case shown="No Error" w393 {
        tunnel: w377 -> [w434 _]
        tunnel: w381 -> [w431 _]
        tunnel: w370 -> [w432 _]
        tunnel: w378 -> [w430 _]
        tunnel: w373 -> [w429 _]
        tunnel: w372 -> [w428 _]
        tunnel: w371 -> [w427 _]
        frame No Error {
          n207 = Bundle By Name(cluster=w434, "nParent"=0) -> (w433:T2)
          n208 = case shown="Default" w430 {
            tunnel: w432 -> [_ w439]
            tunnel: w429 -> [_ w438]
            tunnel: w428 -> [_ w437]
            tunnel: w427 -> [_ w436]
            frame "FLOAT_FRAME_HIDE" {
            }
            frame Default {
              n209 = case shown="Default" w438 {
                tunnel: w439 -> [w441 w446]
                tunnel: w437 -> [_ w443]
                tunnel: w436 -> [_ w442]
                frame Default {
                  n210 = property class="VI"(reference=w441, "Front Panel.Open"=TRUE ("Front Panel Window:Open")) -> ()  [unwired: 1 in, 2 out]
                }
                frame "Document" {
                  n211 = invoke class="SubPnl" method="Insert VI"(reference=w443, "VI Ref"=w442) -> (error out=w444:errorcluster)  [unwired: 2 in, 3 out]
                  n212 = property class="VI"(reference=w446, error in=w444, "Front Panel.Open"=TRUE ("Front Panel Window:Open")) -> ()  [unwired: 2 out]
                }
              }
            }
          }
          n213 = local write "tFrame_Out"(w433) -> ()
          n214 = local write "tSpliter_Out"(w431) -> ()
        }
        frame Error {
        }
      }
    }
    frame "TAB_FRAME", "WIN_FRAME" {
      n215 = case shown="\"TAB_FRAME\", Default" w451 {
        tunnel: w452 -> [w473 w495]
        tunnel: [w467 w501] -> w453
        frame "TAB_FRAME", Default {
          n216 = Unbundle By Name(w473) -> ("pVIF"=w460:refnum<vi>, "pSPW"=w457:refnum<vi>)
          n217 = call "CRYAPI LOAD.vi"("sAction"="LOAD_TAB") -> ("tWindow_Out"=w474:T5)  [unwired: 5 in, 5 out]
          n218 = invoke class="SubPnl" method="Remove VI"(reference=w457) -> (reference out=w463:refnum<vi>, error out=w464:errorcluster)  [unwired: 2 in, 1 out]
          n219 = property class="SubPnl"(reference=w457, "Visible"=FALSE) -> ()  [unwired: 1 in, 2 out]
          n220 = Unbundle By Name(w474) -> ("pVI"=w455:refnum<vi>, "pSP"=w472:refnum<vi>, "pTab"=w470:refnum<vi>, "pSPT"=w465:refnum<vi>)
          n221 = case shown="No Error" w464 {
            selector: w464 -> [w485 w487]
            tunnel: w463 -> [w484 w488]
            tunnel: [w485 w487] -> w461
            tunnel: [w484 w488] -> w462
            tunnel: w460 -> [w483 _]
            frame No Error {
              n222 = call "CRYGet Window Temp Reference.vi"("pVIRef_In"=w483, "sAction"="CLOSE") -> ()  [unwired: 2 in, 8 out]
            }
            frame Error {
            }
          }
          n223 = Bundle By Name(cluster=w473, "pVIF"=w455, "pSPF"=w472, "pTab"=w470, "pSPT"=w465, "nTypeF"=1) -> (w467:T2)
          n224 = Unbundle By Name(w467) -> ("pVIF"=w468:refnum<vi>, "nID"=w469:i32)
          n225 = while {
            tunnel: w455 -> [w481]
            tunnel: [w476] -> w454
            stop <- w477 stop-if-true
            n226 = invoke class="VI" method="Ctrl Val.Get"(reference=w481, "Control Name"="StateOut") -> (reference out=w476:refnum<vi>, "Get Control Value Variant"=w478:variant)  [unwired: 2 in, 2 out]
            n227 = Wait (ms)(milliseconds to wait=u32 10) -> ()  [unwired: 1 out]
            n228 = Variant To Data(type=TRUE, Variant=w478) -> (data=w477:bool)  [unwired: 1 in, 1 out]
          }
          n229 = invoke class="SubPnl" method="Insert VI"(reference=w462, error in=w461, "VI Ref"=w454) -> (reference out=w459:refnum<vi>, error out=w458:errorcluster)  [unwired: 1 in, 2 out]
          n230 = invoke class="VI" method="Ctrl Val.Set"(reference=w468, "Control Name"="WID", "Value"=w469) -> ()  [unwired: 2 in, 5 out]
          n231 = invoke class="SubPnl" method="FitControlToPane"(reference=w459, error in=w458) -> ()  [unwired: 1 in, 3 out]
        }
        frame "WIN_FRAME" {
          n232 = Unbundle By Name(w495) -> ("pVIF"=w491:refnum<vi>, "nTypeF"=w494:i32, "pSPW"=w506:refnum<vi>)
          n233 = invoke class="SubPnl" method="Remove VI"(reference=w506) -> (reference out=w490:refnum<vi>, error out=w505:errorcluster)  [unwired: 2 in, 1 out]
          n234 = call "CRYAPI LOAD.vi"("sAction"="LOAD_EMPTY") -> ("tWindow_Out"=w499:T5)  [unwired: 5 in, 5 out]
          n235 = Equal?(x=1, y=w494) -> (x = y?=w492:bool)
          n236 = Unbundle By Name(w499) -> ("pVI"=w502:refnum<vi>, "pSP"=w498:refnum<vi>, "pTab"=w497:refnum<vi>, "pSPT"=w496:refnum<vi>)
          n237 = case shown="True" w492 {
            tunnel: w491 -> [_ w516]
            tunnel: w490 -> [_ w514]
            tunnel: [_ w514] -> w489
            frame False {
            }
            frame True {
              n238 = call "CRYAPI Get Boolean Reference.vi"("Label Name"="bStop", "VI Refnum"=w516) -> ("Boolean"=w520:bool, "Boolean Ref"=w518:refnum<vi>)  [unwired: 8 out]
              n239 = case shown="True" w520 {
                tunnel: w518 -> [_ w524]
                tunnel: [w521 w522] -> w515
                tunnel: w516 -> [w521 w522]
                frame False {
                }
                frame True {
                  n240 = property class="Bool"(reference=w524, "Val(Sgnl)"=TRUE) -> ()  [unwired: 1 in, 2 out]
                }
              }
              n241 = call "CRYGet Window Temp Reference.vi"("pVIRef_In"=w515, "sAction"="CLOSE") -> ()  [unwired: 2 in, 8 out]
            }
          }
          n242 = invoke class="SubPnl" method="Insert VI"(reference=w490, error in=w505, "VI Ref"=w502) -> (reference out=w504:refnum<vi>, error out=w503:errorcluster)  [unwired: 1 in, 2 out]
          n243 = invoke class="SubPnl" method="FitControlToPane"(reference=w504, error in=w503) -> ()  [unwired: 1 in, 3 out]
          n244 = stacked-sequence {
            tunnel: w502 -> [w513]
            tunnel: [w512] -> w501
            tunnel: w498 -> [w511]
            tunnel: w497 -> [w509]
            tunnel: w496 -> [w508]
            tunnel: w495 -> [w507]
            tunnel: w489 -> [_]
            frame #0 {
              n245 = Bundle By Name(cluster=w507, "pVIF"=w513, "pSPF"=w511, "pTab"=w509, "pSPT"=w508, "nTypeF"=0) -> (w512:T2)
            }
          }
        }
      }
      n246 = local write "tFrame_Out"(w453) -> ()
    }
    frame "CHANGE_PAGE" {
      n247 = Unbundle By Name(w526) -> ("nIDPages"=w533:i32[], "cPages"=w532:T4, "pSPF"=w531:refnum<vi>, "pSPT"=w527:refnum<vi>)
      n248 = Search 1D Array(1D array=w533, element=w534) -> (index of element=w529:i32)  [unwired: 1 out]
      n249 = Not Equal?(x=-1, y=w529) -> (x != y?=w530:bool)
      n250 = case shown="True" w530 {
        tunnel: w529 -> [w536 w540]
        tunnel: w532 -> [w537 w541]
        tunnel: w531 -> [_ w548]
        tunnel: [w537 w543] -> _
        tunnel: [w536 w542] -> _
        tunnel: w527 -> [_ w547]
        tunnel: [0 ("nID") w538] -> w525
        frame False {
        }
        frame True {
          n251 = Index Array(array=w541, index=w540) -> (element=w549:T12)
          n252 = Unbundle By Name(w549) -> ("pVI"=w551:refnum<vi>, "nID"=w539:i32)
          n253 = invoke class="SubPnl" method="Insert VI"(reference=w548, "VI Ref"=w551) -> (reference out=w544:refnum<vi>, error out=w550:errorcluster)  [unwired: 2 in, 2 out]
          n254 = property class="SubPnl"(reference=w547) -> (reference out=w545:refnum<vi>, "Visible"=w546:bool)  [unwired: 1 in, 1 out]
          n255 = case shown="No Error" w550 {
            tunnel: w549 -> [w555 w567]
            tunnel: [w555 w567] -> _
            tunnel: w546 -> [w558 _]
            tunnel: w545 -> [w557 _]
            tunnel: w544 -> [w556 _]
            tunnel: [w554 w566] -> w543
            tunnel: w541 -> [w554 w566]
            tunnel: [w553 w565] -> w542
            tunnel: w540 -> [w553 w565]
            tunnel: [w552 0 ("nID")] -> w538
            tunnel: w539 -> [w552 _]
            frame No Error {
              n256 = case shown="True" w558 {
                tunnel: w557 -> [_ w563]
                tunnel: w556 -> [_ w560]
                tunnel: [_ w559] -> _
                frame False {
                }
                frame True {
                  n257 = property class="SubPnl"(reference=w563, "Visible"=FALSE) -> ()  [unwired: 1 in, 2 out]
                  n258 = property class="SubPnl"(reference=w560, "Visible"=TRUE) -> (reference out=w559:refnum<vi>)  [unwired: 1 in, 1 out]
                }
              }
            }
            frame Error {
            }
          }
        }
      }
      n259 = local write "nData_Out"(w525) -> ()
    }
    frame "FIND_WIN", "FIND_WIN_ID", "FIND_WIN_STEMP", "FIND_WIN_TITLE" {
      n260 = case shown="\"FIND_WIN\", \"FIND_WIN_STEMP\"" w569 {
        tunnel: w574 -> [_ w590 w602]
        tunnel: [w575 w592 w604] -> w573
        tunnel: [w577 w591 w603] -> w571
        tunnel: w568 -> [w576 _ _]
        frame "FIND_WIN_ID", Default {
          n261 = global read "CRYMain Sub Window Global.vi" "cFrame"() -> (w581:T6)
          n262 = Unbundle By Name(w581) -> ("nID"=w580:i32[], "Frame"=w578:T7)
          n263 = Search 1D Array(1D array=w580, element=w576) -> (index of element=w579:i32)  [unwired: 1 out]
          n264 = case shown="-1" w579 {
            selector: w579 -> [w584 _]
            tunnel: w578 -> [w585 _]
            tunnel: [w583 T2 {"nType"=0, "nParent"=0, "pVIW"=refnum, "pSPW"=refnum, "nTypeF"=0, "pVIF"=refnum, "pSPF"=refnum, "nIDSpliter"=0, "nProperty"=0, "Bound"={"Left"=0, "Top"=0, "Right"=0, "Bottom"=0}, "nID"=0, "nData"=0, "sData"="", "pWVI"=refnum, "sTitle"="", "cPages"=[], "pTab"=refnum, "nIDPages"=[], "pSPT"=refnum, "sTemp"="", "nDockID"=0, "nDockLR"=0, "sIcon"=""} ("tFrame_Out")] -> w577
            tunnel: w576 -> [w582 _]
            tunnel: [w582 0 ("nData")] -> w575
            frame Default {
              n265 = Index Array(array=w585, index=w584) -> (element=w583:T2)
            }
            frame -1 {
            }
          }
        }
        frame "FIND_WIN", "FIND_WIN_STEMP" {
          n266 = global read "CRYMain Sub Window Global.vi" "cFrame"() -> (w589:T6)
          n267 = Unbundle By Name(w589) -> ("Frame"=w588:T7)
          n268 = for {
            tunnel: w588 -> [w597] mode=indexing
            tunnel: w590 -> [w598]
            tunnel: [w597] -> w591
            tunnel: [w593] -> w592
            stop <- w596 stop-if-true
            n269 = Unbundle By Name(w597) -> ("sTemp"=w599:string, "nID"=w595:i32)
            n270 = Equal?(x=w599, y=w598) -> (x = y?=w596:bool)
            n271 = Select(t=w595, s=w596, f=0) -> (s? t:f=w593:i32)
          }
        }
        frame "FIND_WIN_TITLE" {
          n272 = global read "CRYMain Sub Window Global.vi" "cFrame"() -> (w601:T6)
          n273 = Unbundle By Name(w601) -> ("Frame"=w600:T7)
          n274 = for {
            tunnel: w600 -> [w609] mode=indexing
            tunnel: w602 -> [w610]
            tunnel: [w609] -> w603
            tunnel: [w605] -> w604
            stop <- w608 stop-if-true
            n275 = Unbundle By Name(w609) -> ("sTitle"=w611:string, "nID"=w607:i32)
            n276 = Equal?(x=w611, y=w610) -> (x = y?=w608:bool)
            n277 = Select(t=w607, s=w608, f=0) -> (s? t:f=w605:i32)
          }
        }
      }
      n278 = local write "tFrame_Out"(w571) -> ()
      n279 = local write "nData_Out"(w573) -> ()
      n280 = Greater Than 0?(x=w573) -> (x > 0?=w572:bool)
      n281 = case shown="True" w572 {
        tunnel: w571 -> [_ w617]
        tunnel: ["NOT FOUND" w615] -> w570
        frame False {
        }
        frame True {
          n282 = Unbundle By Name(w617) -> ("nParent"=w613:i32, "pVIW"=w616:refnum<vi>)
          n283 = Equal To 0?(x=w613) -> (x = 0?=w614:bool)
          n284 = case shown="True" w614 {
            tunnel: w616 -> [_ w623]
            tunnel: ["OPEN" w619] -> w615
            frame False {
            }
            frame True {
              n285 = property class="VI"(reference=w623) -> ("Front Panel.Open"=w621:bool)  [unwired: 1 in, 2 out]
              n286 = Select(t="OPEN", s=w621, f="CLOSE") -> (s? t:f=w619:string)
            }
          }
        }
      }
      n287 = local write "sData_Out"(w570) -> ()
    }
    frame "RECOVERY_FRAME" {
      # "Recovery User VI Data"
      n288 = Unbundle By Name(w628) -> ("pSPF"=w627:refnum<vi>, "pWVI"=w626:refnum<vi>)
      n289 = invoke class="SubPnl" method="Insert VI"(reference=w627, "VI Ref"=w626) -> (reference out=w625:refnum<vi>, error out=w624:errorcluster)  [unwired: 2 in, 2 out]
      n290 = invoke class="SubPnl" method="FitControlToPane"(reference=w625, error in=w624) -> ()  [unwired: 1 in, 3 out]
      n291 = local write "tFrame_Out"(w628) -> ()
    }
    frame "GetFrameType" {
      n292 = Unbundle By Name(w641) -> ("nTypeF"=w664:i32)
      n293 = Unbundle By Name(w641) -> ("sTemp"=w648:string)
      n294 = Unbundle By Name(w641) -> ("nType"=w667:i32)
      n295 = Unbundle By Name(w641) -> ("sTemp"=w633:string)
      n296 = Unbundle By Name(w641) -> ("sTemp"=w646:string)
      n297 = Equal?(x=w667, y=1) -> (x = y?=w662:bool)
      n298 = Equal?(x=w664, y=0) -> (x = y?=w661:bool)
      n299 = Equal?(x=w648, y="Step Setup") -> (x = y?=w652:bool)
      n300 = Equal?(x=w646, y="Document") -> (x = y?=w643:bool)
      n301 = Equal?(x=w633, y="StepView") -> (x = y?=w634:bool)
      n302 = Equal?(x=w633, y="DataView") -> (x = y?=w635:bool)
      n303 = Equal?(x=w633, y="ResultView") -> (x = y?=w636:bool)
      n304 = Match Pattern(string=w633, regular expression="StepView") -> (offset past match=w631:i32)  [unwired: 1 in, 3 out]
      n305 = Compound Arithmetic op=AND(w662, w661) -> (w660:bool)
      n306 = Not Equal?(x=w631, y=-1) -> (x != y?=w629:bool)
      n307 = Select(t=200 ("y"), s=w652, f=0 ("y")) -> (s? t:f=w647:i32)
      n308 = Select(t=1000 ("y"), s=w660, f=0 ("y")) -> (s? t:f=w655:i32)
      n309 = Select(t=10 ("y"), s=w643, f=0 ("y")) -> (s? t:f=w642:i32)
      n310 = Compound Arithmetic op=OR(w634, w635, w636, w629) -> (w637:bool)
      n311 = Select(t=100 ("y"), s=w637, f=0 ("y")) -> (s? t:f=w654:i32)
      n312 = Compound Arithmetic op=ADD(w655, w654, w647, w642) -> (w653:i32)
      n313 = case shown="1010" w653 {
        frame Default {
          n314 = local write "sData_Out"("FRAME" ("sData_Out")) -> ()
        }
        frame 1100 {
          # "WINDOW+WINDOW+VIEW"
          n315 = local write "sData_Out"("FRAME_VIEW" ("sData_Out")) -> ()
        }
        frame 1200 {
          # "WINDOW+WINDOW+VIEW"
          n316 = local write "sData_Out"("FRAME_STEP" ("sData_Out")) -> ()
        }
        frame 1010 {
          # "WINDOW+WINDOW+VIEW"
          n317 = local write "sData_Out"("FRAME_DOCUMENT" ("sData_Out")) -> ()
        }
      }
    }
  }
